vi "Read Status.vi"(8 "error in (no error)":errorcluster, 11 "Customer in":refnum<class "Customer.lvclass">) -> (0 "error out":errorcluster, 2 "Status":string, 3 "Customer out":refnum<class "Customer.lvclass">)   [LabVIEW 2023, in "Customer.lvlib" / "Customer.lvclass"]
doc: "Returns the customer's current status. This status is displayed in the top-level coffee shop's user interface."
uses:
  Customer.lvclass
  Customer.lvclass/Customer.ctl
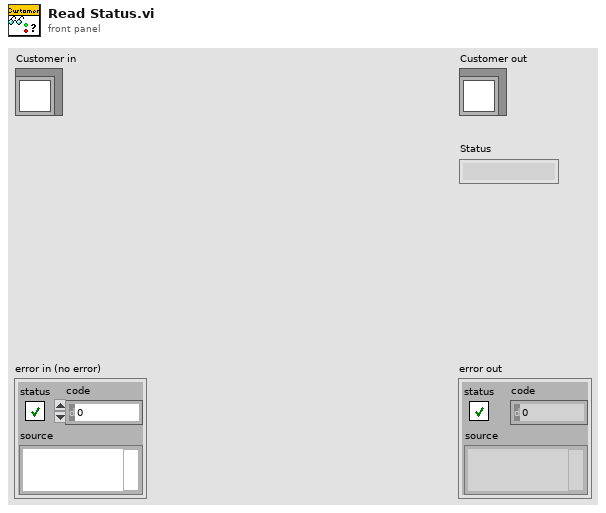
[diagram p1: front panel]
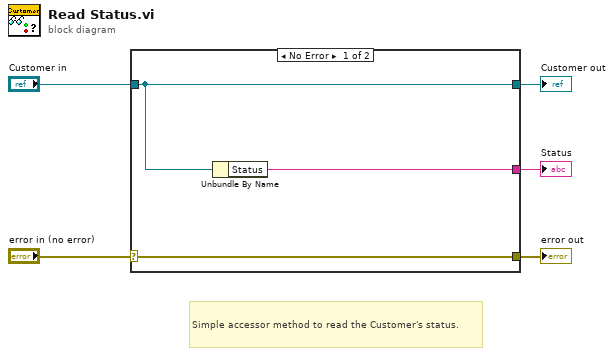
[diagram p0: block diagram]
diagram:
  # "Simple accessor method to read the Customer's status."
  n1 = case shown="No Error" "error in (no error)" {
    selector: "error in (no error)" -> [w8 w9]
    tunnel: [w8 w9] -> w4
    tunnel: [w7 w10] -> w2
    tunnel: "Customer in" -> [w7 w10]
    tunnel: [w6 _] -> w1
    frame No Error {
      n2 = Unbundle By Name(w7) -> ("Status"=w6:string)
    }
    frame Error {
    }
  }
  "error out" <- w4
  "Customer out" <- w2
  "Status" <- w1
